vi "Test_Aquisition_Reactor_Coolant_Loop Temperature_SG_Inlet_Average.vi"() -> ()   [LabVIEW 2022 SP3]
uses:
  SI_modules/SI101/SI101.lvclass
panel:
  out "Avg Temp rise":cluster{"Time":timestamp[], dbl[]}[](graph)
  out "Inputs":cluster{"Time":timestamp[], dbl[]}[](graph)
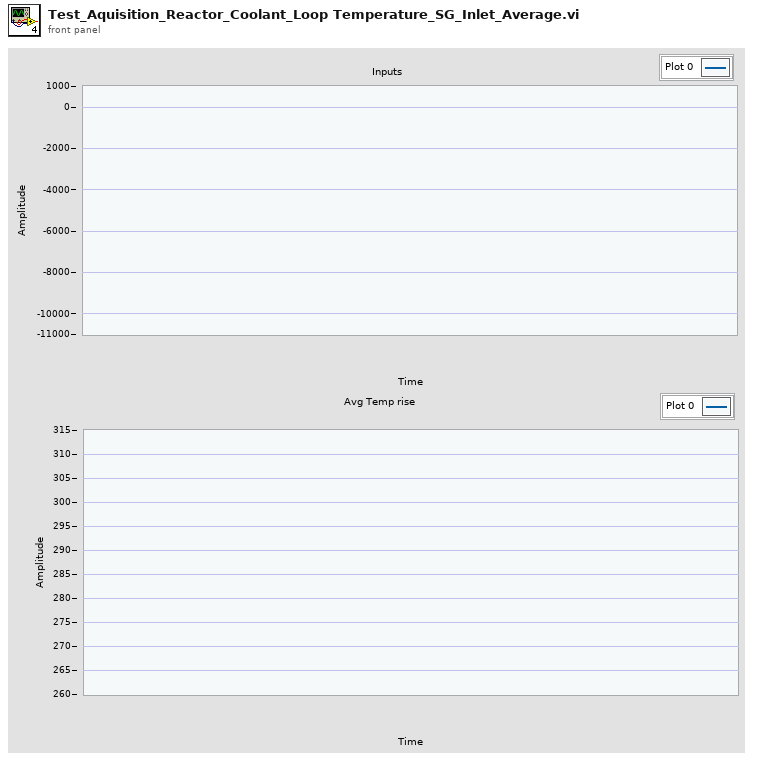
[diagram p1: front panel]
types:
  T1 = cluster{"[0]":cluster{"Time":timestamp[], "KKS":string, "Meas":dbl[]}, "[1]":cluster{"Time":timestamp[], "KKS":string, "Meas":dbl[]}, "[2]":cluster{"Time":timestamp[], "KKS":string, "Meas":dbl[]}, "[3]":cluster{"Time":timestamp[], "KKS":string, "Meas":dbl[]}, "[4]":cluster{"Time":timestamp[], "KKS":string, "Meas":dbl[]}, "[5]":cluster{"Time":timestamp[], "KKS":string, "Meas":dbl[]}, "[6]":cluster{"Time":timestamp[], "KKS":string, "Meas":dbl[]}, "[7]":cluster{"Time":timestamp[], "KKS":string, "Meas":dbl[]}, "[8]":cluster{"Time":timestamp[], "KKS":string, "Meas":dbl[]}}
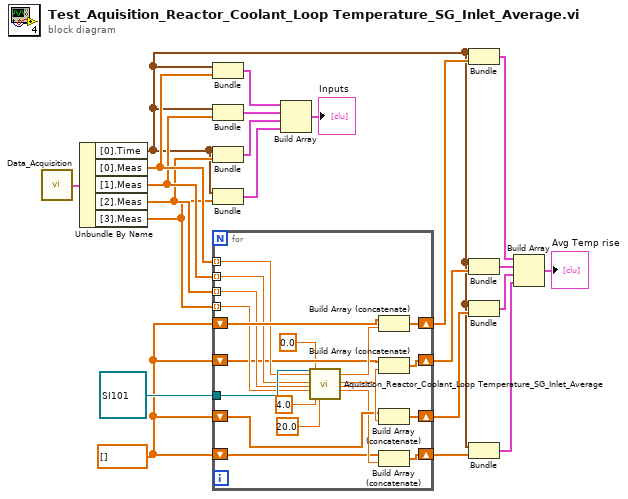
[diagram p0: block diagram]
diagram:
  w11 = dbl[] []
  n1 = call "Data_Acquisition.vi"() -> ("Meas"=w22:T1)  [unwired: 15 in]
  n2 = Unbundle By Name(w22) -> ("[0].Time"=w1:timestamp[], "[0].Meas"=w21:dbl[], "[1].Meas"=w20:dbl[], "[2].Meas"=w19:dbl[], "[3].Meas"=w18:dbl[])
  n3 = Bundle("Time"=w1, "Meas"=w21) -> (w17:cluster{"Time":timestamp[], "Meas":dbl[]})  [unwired: 1 in]
  n4 = Bundle("Time"=w1, "Meas"=w20) -> (w16:cluster{"Time":timestamp[], "Meas":dbl[]})  [unwired: 1 in]
  n5 = Bundle("Time"=w1, "Meas"=w19) -> (w15:cluster{"Time":timestamp[], "Meas":dbl[]})  [unwired: 1 in]
  n6 = Bundle("Time"=w1, "Meas"=w18) -> (w14:cluster{"Time":timestamp[], "Meas":dbl[]})  [unwired: 1 in]
  n7 = for {
    tunnel: w21 -> [w40] mode=indexing
    tunnel: w20 -> [w39] mode=indexing
    tunnel: w19 -> [w38] mode=indexing
    tunnel: w18 -> [w37] mode=indexing
    shift-right: [w30] -> w2
    shift-left: w11 -> [w42]
    tunnel: refnum<class "SI101.lvclass"> refnum ("SI101_AverageReactorCoolantTemperature.lvclass") -> [w41]
    shift-right: [w31] -> w10
    shift-left: w11 -> [w32]
    shift-right: [w28] -> w9
    shift-left: w11 -> [w27]
    shift-right: [w25] -> w8
    shift-left: w11 -> [w24]
    n8 = call "Aquisition_Reactor_Coolant_Loop Temperature_SG_Inlet_Average.vi"("SI101_AverageReactorCoolantTemperature.lvclass"=w41, "3 JEC10 CT001B XQ01"=w40, "3 JEC20 CT001B XQ01"=w39, "3 JEC30 CT001B XQ01"=w38, "3 JEC40 CT001B XQ01"=w37, "SI100 Avg Temp Rise"=0.0, "In1"=4.0, "In2"=20.0) -> ("ACT Loop 1"=w34:dbl, "ACT Loop 2"=w33:dbl, "ACT loop 3"=w29:dbl, "ACT loop 4"=w26:dbl)  [unwired: 14 in, 2 out]
    n9 = Build Array (concatenate)(w42, w34) -> (w30:dbl[])
    n10 = Build Array (concatenate)(w32, w33) -> (w31:dbl[])
    n11 = Build Array (concatenate)(w27, w29) -> (w28:dbl[])
    n12 = Build Array (concatenate)(w24, w26) -> (w25:dbl[])
  }
  n13 = Build Array(w17, w16, w15, w14) -> (→"Inputs":cluster{"Time":timestamp[], "Meas":dbl[]}[])
  n14 = Bundle("Time"=w1, w2) -> (w3:cluster{"Time":timestamp[], dbl[]})  [unwired: 1 in]
  n15 = Bundle("Time"=w1, w10) -> (w7:cluster{"Time":timestamp[], dbl[]})  [unwired: 1 in]
  n16 = Bundle("Time"=w1, w9) -> (w6:cluster{"Time":timestamp[], dbl[]})  [unwired: 1 in]
  n17 = Bundle("Time"=w1, w8) -> (w5:cluster{"Time":timestamp[], dbl[]})  [unwired: 1 in]
  n18 = Build Array(w3, w7, w6, w5) -> (→"Avg Temp rise":cluster{"Time":timestamp[], dbl[]}[])
